vi "HS_ConvertSize.vi"(11 "read buffer":string) -> (2 "# bytes":u32, 3 "size()":u32[](array[numeric]))   [LabVIEW 2019]
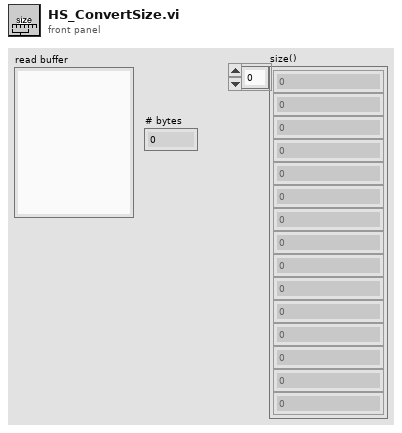
[diagram p1: front panel]
types:
  T1 = enum16{"big-endian, network order", "native, host order", "little-endian"}
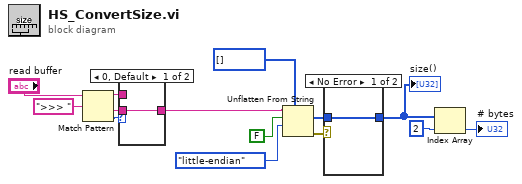
[diagram p0: block diagram]
diagram:
  n1 = Match Pattern(string="read buffer", regular expression=">>> ") -> (before substring=w4:string, after substring=w3:string, offset past match=w5:i32)  [unwired: 1 in, 1 out]
  n2 = case shown="0, Default" w5 {
    tunnel: [w15 w16] -> w1
    tunnel: w4 -> [_ w16]
    tunnel: w3 -> [w15 _]
    frame 0, Default {
    }
    frame -1 {
    }
  }
  n3 = Unflatten From String(type=u32[] [], binary string=w1, data includes array or string size? (T)=FALSE, byte order (0:big-endian, network order)=T1."little-endian") -> (value=w7:u32[], error out=w9:errorcluster)  [unwired: 1 in, 1 out]
  n4 = case shown="No Error" w9 {
    tunnel: [w17 _] -> w8
    tunnel: w7 -> [w17 _]
    frame No Error {
    }
    frame Error {
    }
  }
  "size()" <- w8
  n5 = Index Array(array=w8, index=2) -> (element=→"# bytes":u32)
